vi "Lidar V2 RT Main.vi"() -> ()   [LabVIEW 2013]
uses:
  <vilib>/FPGAPlugInAG/PXIe-7962R/niLvFpga_Open_PXIe-7962R.vi
  <vilib>/rvi/interface/common/dynamic/niFpgaDynamicAddResources.vi
  <vilib>/FPGAPlugInAG/Dynamic/niLvFpga_Abort_Dynamic.vi
  <vilib>/FPGAPlugInAG/Dynamic/niLvFpga_Reset_Dynamic.vi
  <vilib>/FPGAPlugInAG/Dynamic/niLvFpga_Run_Dynamic.vi
  <vilib>/rvi/interface/common/niFpgaWaitOnOcc.vi
  <vilib>/Utility/error.llb/Error Cluster From Error Code.vi
  <vilib>/rvi/errors/niLvFpgaAdjustHostInterfaceError.vi
  <vilib>/FPGAPlugInAG/Dynamic/niLvFpga_Close_Dynamic.vi
  <vilib>/rvi/interface/nirviOpenFPGA/nirviOpenFPGA.xnode
  FPGA Bitfiles/LIDAR Module 5782 V5.9.lvbitx
  <vilib>/rvi/interface/nirviMethod/nirviMethod.xnode
  <vilib>/rvi/interface/nirviReadWriteControl/nirviReadWriteControl.xnode
  <vilib>/rvi/interface/nirviCloseFPGA/nirviCloseFPGA.xnode
  <vilib>/FPGAPlugInAG/Dynamic/niLvFpga_ReadFifo_Dynamic.vi
  <vilib>/rvi/errors/niLvFpgaMergeErrorWithErrorCode.vi
  <vilib>/ptbypt/NI_PtbyPt.lvlib
  <vilib>/Analysis/NI_AALBase.lvlib
  NiFpgaLv.dll
  <vilib>/rvi/interface/Simulation/niFpgaSimulationCallBeginRW.vi
panel:
  in  "MaxStartSample":u8=54
  out "Intensity Map":u32[][](graph)=[[38267, 40863, 43426, 46903, 50379, 49577, 9511, 20052, 7258, 36545, 49622, 30765, 7679, 11446, 11287, 8610], [45519, 42398, 47961, 47044, 51202, 50615, 46477, 39458, 9841, 41698, 52891, 31717, 7088, 8130, 9027, 8119], [48671, 50114, 49333, 52463, 55996, 55598, 55499, 50228, 23748, 32917, 46824, 34677, 16354, 12518, 13710, 14465], [54064, 48927, 52198, 54292, 54548, 47730, 56020, 55390, 37937, 50069, 55178, 34706, 86530, 9874, 15467, 8958], [54127, 52666, 53875, 65066, 101095, 130103, 75733, 59949, 29491, 65502, 50785, 24349, 16198, 8817, 5686, 6636], [63717, 51110, 54640, 82482, 144722, 130520, 117220, 19151, 20018, 18186, 19523, 16677, 18204, 12359, 7312, 6192], [60324, 57984, 72516, 113653, 133185, 141195, 138982, 19785, 13914, 20568, 17572, 18332, 36391, 16559, 8656, 7239], [10675, 84263, 85858, 130204, 147736, 162189, 159832, 21467, 21876, 17164, 11455, 43385, 116640, 15279, 7969, 6867], [37695, 141137, 100147, 149060, 144081, 168934, 167216, 19438, 20260, 21484, 18662, 15530, 119323, 10502, 5990, 5756], [69488, 62058, 50045, 120398, 134387, 151104, 149833, 157001, 47922, 18908, 19123, 19272, 18373, 18944, 18110, 15447], [59157, 62414, 58749, 57578, 60555, 55810, 53103, 60527, 53706, 145306, 42304, 18833, 19783, 8385, 18856, 18720], [64249, 59919, 59597, 60756, 61047, 63017, 64938, 58053, 10510, 155082, 62144, 37988, 7375, 10245, 16147, 15414], [62678, 57333, 55641, 62329, 59085, 64488, 62926, 68318, 5831, 27753, 56193, 49801, 7109, 11185, 14695, 13534], [64860, 57918, 61295, 61918, 64011, 61837, 64216, 68709, 45145, 38007, 52474, 54336, 122862, 23649, 16487, 16877], [64466, 54840, 60724, 63188, 59161, 63167, 61944, 113757, 46296, 65445, 86895, 55833, 117827, 25177, 22545, 24674], [63747, 55429, 56781, 62403, 60957, 62337, 68183, 109145, 46415, 64989, 46515, 60255, 95561, 24349, 18046, 19264], [59827, 54805, 52448, 56788, 59923, 57562, 61463, 61241, 41494, 17316, 22198, 36981, 63082, 17749, 12719, 12336], [55570, 53617, 51599, 51841, 54806, 55615, 59827, 59503, 38863, 55313, 57948, 58576, 79827, 20327, 14840, 15093], [52952, 51728, 52895, 50260, 50904, 54415, 56882, 53800, 42244, 17470, 32064, 64825, 52564, 15197, 14516, 13645], [45412, 46585, 49451, 49892, 46454, 50593, 66473, 70481, 31893, 54244, 80137, 82405, 102857, 102147, 33680, 28535]]
  in  "10thIndexDeb":u8
  in  "ActiveLedIndexDeb":u16
  in  "LedScanDebEn":bool
  out "Numeric":i32=1666
  in  "LaserPower 1":bool=TRUE
  in  "LaserPower 0":bool=TRUE
  out "median":dbl=92741.0 format="%0.2f"
  out "Range Map":u32[][](graph)=[[93610, 93475, 93265, 93026, 92936, 93011, 90522, 93400, 92936, 93355, 93340, 93086, 91182, 91587, 91437, 91437], [93385, 93370, 93250, 93205, 93041, 92936, 92666, 93131, 91976, 93280, 93190, 93250, 92441, 92336, 91811, 91437], [93550, 93445, 93026, 92726, 92576, 92321, 92471, 93385, 93146, 93101, 93086, 93101, 95934, 92681, 86595, 86340], [93655, 93595, 93071, 92681, 92531, 89158, 92546, 93325, 92936, 92996, 93190, 93340, 93280, 88993, 86550, 88094], [93460, 93280, 93026, 86940, 86625, 86715, 86745, 91841, 91976, 92306, 93295, 92936, 86760, 86610, 89938, 89938], [93190, 93250, 86565, 86505, 86475, 86370, 86325, 86520, 86505, 86760, 86415, 86580, 86580, 92741, 91437, 89938], [93325, 93190, 86730, 86535, 86445, 86475, 86475, 86670, 86550, 86565, 86430, 86625, 93985, 92756, 90897, 89938], [95829, 86685, 86550, 86460, 86475, 86520, 86580, 86535, 86430, 86580, 92936, 93131, 93175, 92621, 90477, 89938], [93101, 86400, 86160, 86145, 86235, 86280, 86130, 86490, 86385, 86445, 86580, 86940, 93011, 86835, 90118, 89938], [93026, 92861, 92756, 86370, 86265, 86160, 86160, 86115, 86400, 86460, 86400, 86505, 86625, 86490, 86535, 86565], [93220, 93190, 93056, 92771, 92576, 92486, 92501, 92861, 86220, 86070, 86280, 86565, 86550, 88694, 86565, 86460], [93146, 93235, 92786, 92621, 92606, 92621, 92726, 92801, 90537, 92336, 92711, 92726, 96158, 91437, 91317, 91047], [92891, 92771, 92771, 92756, 92801, 92816, 92666, 92696, 91437, 92651, 92816, 92711, 93101, 91856, 91811, 91781], [92936, 92936, 93041, 93011, 92996, 92936, 92936, 92936, 92486, 92936, 92936, 92936, 93041, 92771, 92306, 92126], [93041, 93131, 93026, 92726, 92681, 92666, 92621, 92351, 91856, 91796, 92606, 92756, 92936, 92681, 91871, 91751], [93175, 93161, 92846, 92786, 92726, 92861, 92636, 92216, 91796, 91826, 92816, 92816, 92756, 92441, 91437, 91602], [92936, 92741, 92726, 92756, 92936, 92771, 92741, 92711, 91811, 92591, 92711, 92681, 92726, 92351, 91437, 91766], [92771, 92846, 92861, 92936, 92771, 92711, 92771, 92786, 92111, 92591, 92666, 92786, 92936, 92591, 92216, 91677], [93071, 93086, 93041, 92816, 92741, 92786, 92936, 93056, 91871, 92441, 92606, 92831, 92936, 92516, 91437, 91212], [93026, 92936, 92831, 92711, 92756, 92936, 92426, 92351, 90597, 90612, 90642, 90642, 90447, 90402, 90238, 90223]]
  in  "PulseUpClck":u16=4
  in  "PulseWaitClck":u16=30
  in  "Devider":u8=1
  in  "ScanFormat":enum16{"1PulsePerLed", "FullScanPerLed"}(ring)=enum."FullScanPerLed"
  in  "Freq [Mhz]":dbl=100000000.0 format="%#_6p"
  out "error out":errorcluster
  out "standard deviation":dbl=2806.7231162507614 format="%0.5f"
  out "Coarse":dbl
  out "Fine":dbl
  in  "empty graph data":bool
  out "hi(x) 2":i32[][](graph)
  out "hi(x)":i32[](array[numeric])
  out "interval":u32=4
  in  "y":dbl=57.0
  out "Range":dbl=0.4861031988439848 format="%#.2f"
  out "Distance":dbl=88993.39115730001 format="%#.4f"
  out "mean":dbl=57.486103198843985 format="%0.2f"
  out "Fine":u16[](array[numeric])=[88, 76, 70, 116, 105, 79, 74, 115, 111, 107, 100, 88, 86, 100, 100, 134, 110, 60, 83, 137]
  out "Coarse":u16[](array[numeric])=[57, 57, 62, 61, 61, 57, 57, 63, 61, 61, 61, 61, 61, 61, 61, 59, 60, 61, 61, 58]
  in  "stop":bool=TRUE
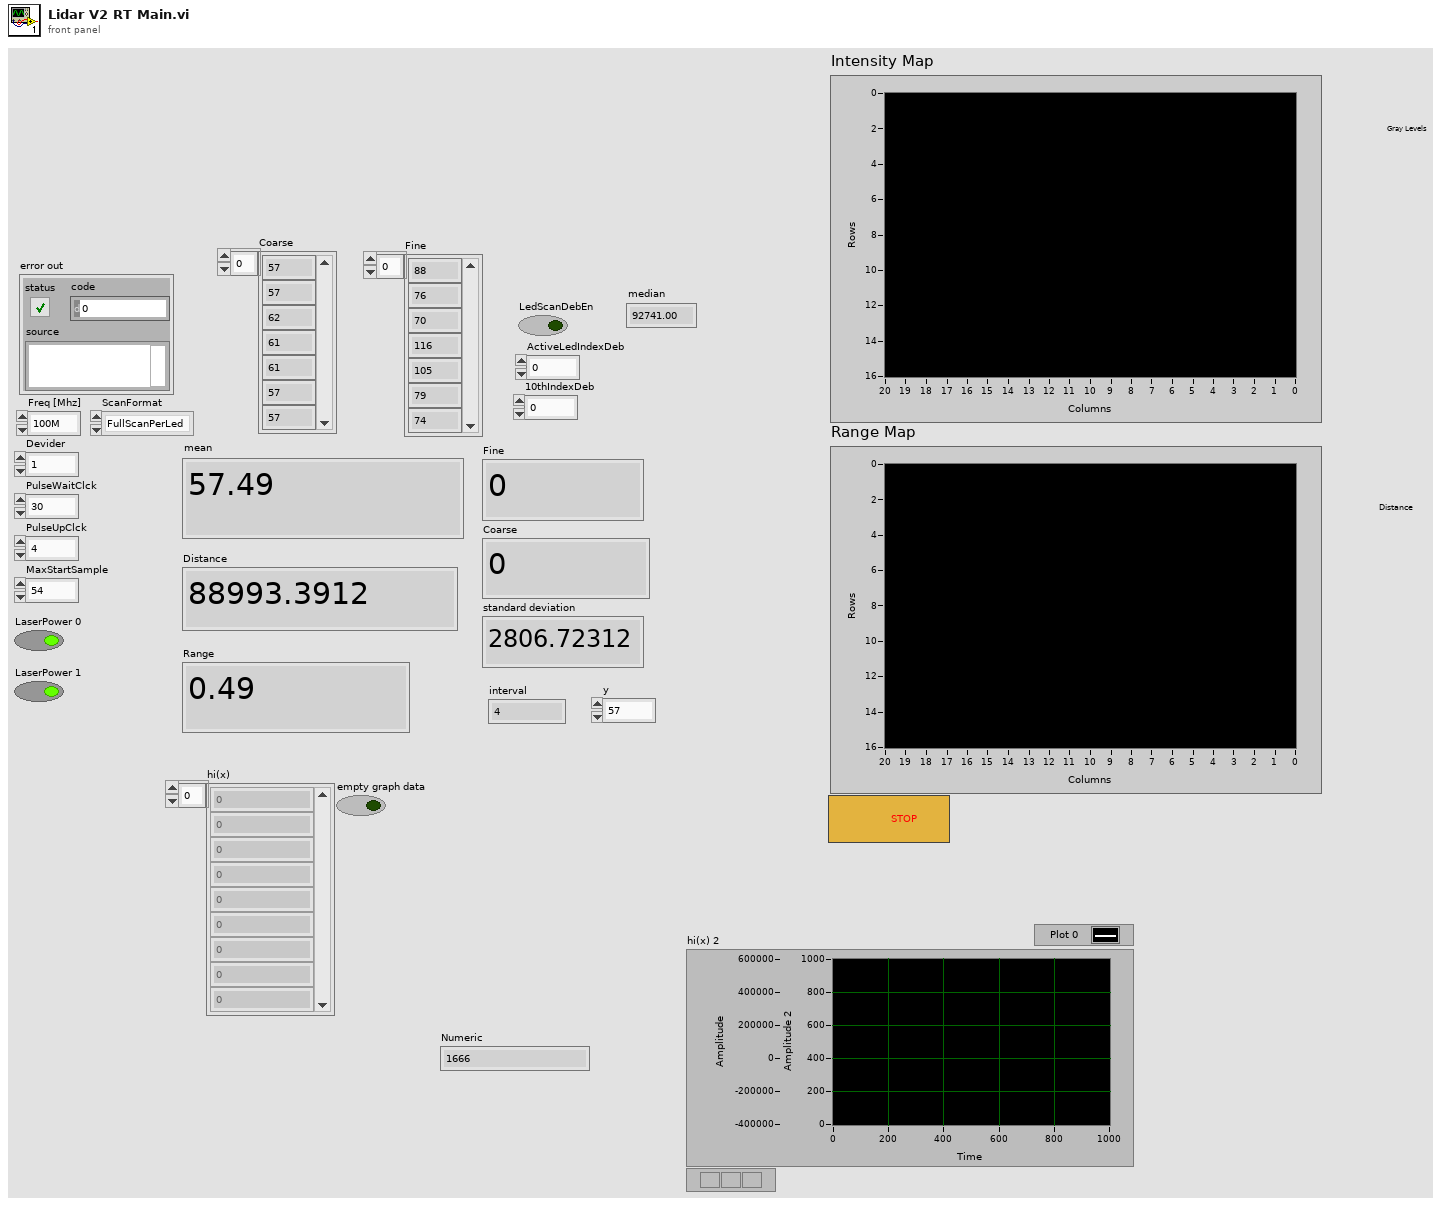
[diagram p1: front panel]
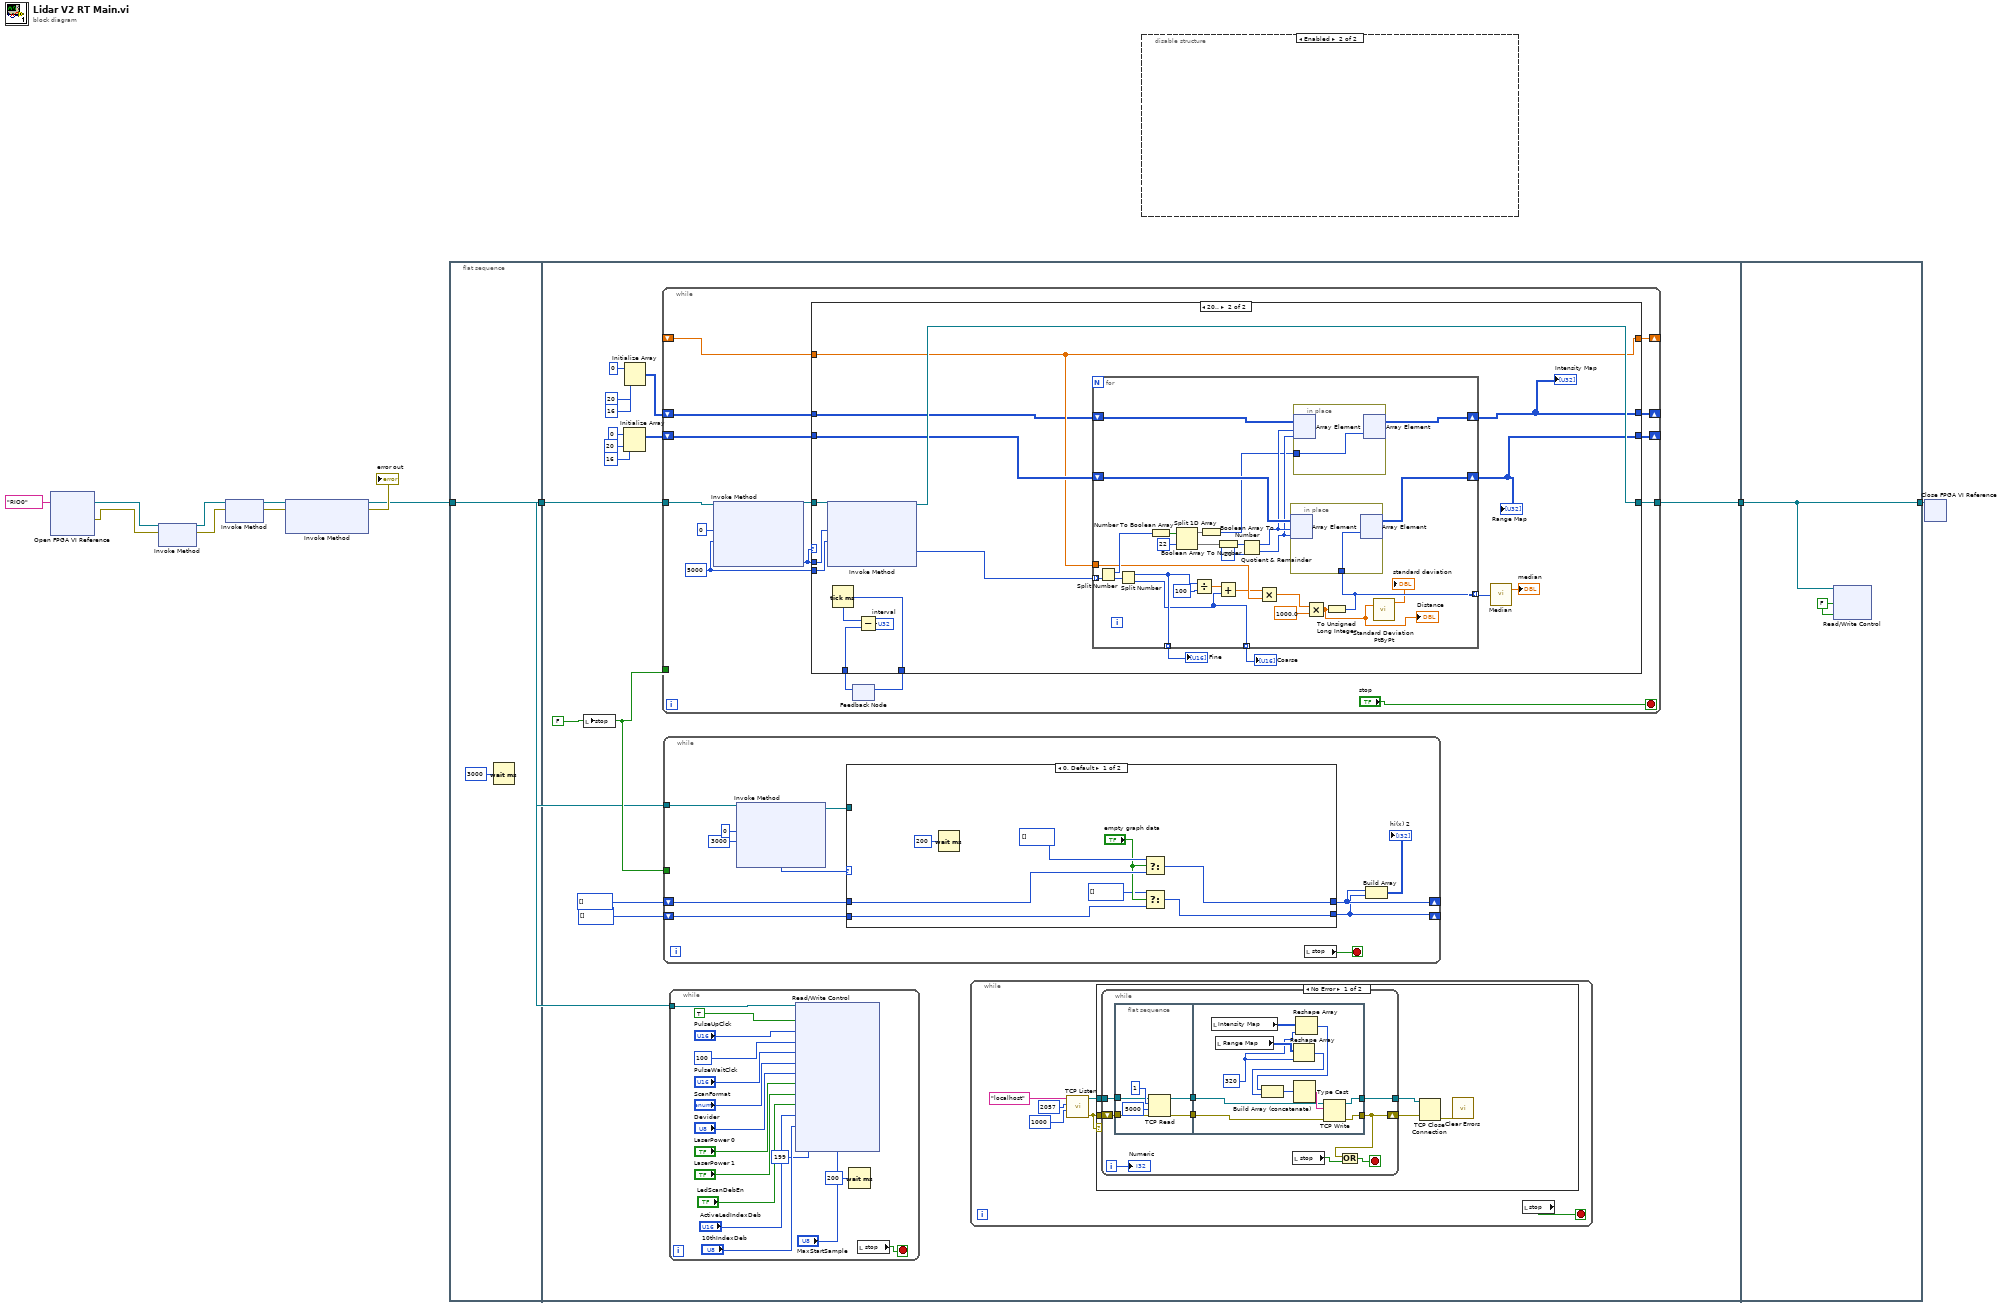
[diagram p0: block diagram]
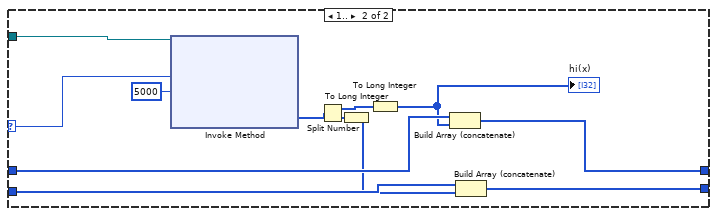
[diagram p3: hidden frame]
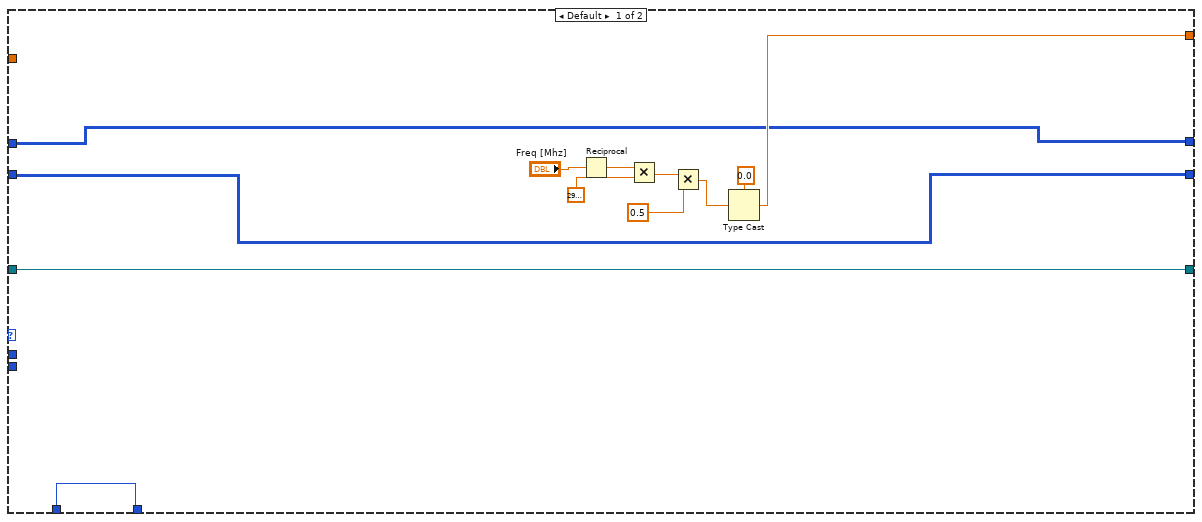
[diagram p4: hidden frame]
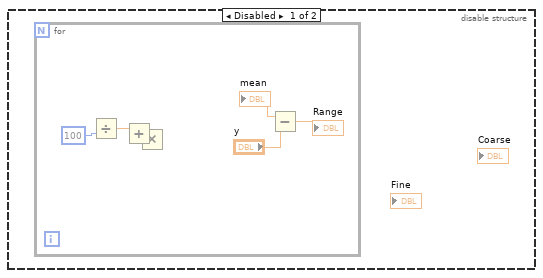
[diagram p5: hidden frame]
diagram:
  n1 = xnode "Open FPGA VI Reference"("resource name"=tag "RIO0") -> ("FPGA VI Reference Out"=w4:refnum<k20>, "error out"=w2:errorcluster)  [unwired: 1 in]
  n2 = xnode "Invoke Method"("FPGA VI Reference In"=w4, "error in"=w2) -> ("FPGA VI Reference Out"=w3:refnum<k20>, "error out"=w1:errorcluster)
  n3 = xnode "Invoke Method"("FPGA VI Reference In"=w3, "error in"=w1) -> ("FPGA VI Reference Out"=w10:refnum<k20>, "error out"=w9:errorcluster)
  n4 = xnode "Invoke Method"("FPGA VI Reference In"=w10, "error in"=w9) -> ("FPGA VI Reference Out"=w7:refnum<k20>, "error out"=→"error out":errorcluster)  [unwired: 1 in]
  n5 = flat-sequence {
    tunnel: w7 -> [w14]
    tunnel: [w14] -> w6
    tunnel: w6 -> [w23]
    tunnel: [w27] -> w5
    tunnel: [w186] -> w11
    tunnel: w5 -> [w186]
    frame #0 {
      n6 = Wait (ms)(milliseconds to wait=u32 3000) -> ()  [unwired: 1 out]
    }
    frame #1 {
      w26 = FALSE ("stop")
      n7 = local write "stop"(w26) -> ()
      n8 = Initialize Array(u32 0 ("element"), 20 ("dimension size"), 16 ("dimension size")) -> (w19:u32[][])
      n9 = Initialize Array(u32 0 ("element"), 20 ("dimension size"), 16 ("dimension size")) -> (w15:u32[][])
      n10 = while {
        tunnel: w23 -> [w126]
        tunnel: [w121] -> w27
        tunnel: w26 -> [_]
        shift-right: [w117] -> _
        shift-left: _ -> [w116]
        shift-right: [w114] -> _
        shift-left: w19 -> [w115]
        shift-right: [w112] -> _
        shift-left: w15 -> [w113]
        stop <- "stop" stop-if-true
        w123 = 5000 ("Timeout (ms)")
        n11 = xnode "Invoke Method"("FPGA VI Reference In"=w126, "Number of Elements"=u32 0, "Timeout (ms)"=w123) -> ("FPGA VI Reference Out"=w124:refnum<k20>, "Elements Remaining"=w120:u32)  [unwired: 1 in, 2 out]
        n12 = feedback #1() -> (w118:u32)  [unwired: 1 in]
        n13 = case shown="20.." w120 {
          tunnel: w124 -> [w138 w155]
          tunnel: w120 -> [_ w154]
          tunnel: w123 -> [_ w153]
          tunnel: [w138 w151] -> w121
          tunnel: [w137 w150] -> w119
          tunnel: w118 -> [w137 w149]
          tunnel: [w129 w146] -> w117
          tunnel: w116 -> [_ w146]
          tunnel: w115 -> [w128 w147]
          tunnel: [w128 w145] -> w114
          tunnel: w113 -> [w127 w140]
          tunnel: [w127 w139] -> w112
          frame Default {
            n14 = Reciprocal(x="Freq [Mhz]") -> (1/x=w136:dbl)
            n15 = Multiply(x=w136, y=dbl[unit] 299792458.0) -> (x*y=w133:dbl[unit])
            n16 = Multiply(x=w133, y=dbl[unit] 0.5) -> (x*y=w130:dbl[unit])
            n17 = Type Cast(type=0.0 ("y"), x=w130) -> (*(type *) &x=w129:dbl)
          }
          frame 20.. {
            n18 = xnode "Invoke Method"("FPGA VI Reference In"=w155, "Number of Elements"=w154, "Timeout (ms)"=w153) -> ("FPGA VI Reference Out"=w151:refnum<k20>, "Data"=w152:u64[])  [unwired: 1 in, 2 out]
            n19 = Tick Count (ms)() -> (millisecond timer value=w150:u32)
            n20 = Subtract(x=w150, y=w149) -> (x-y=→"interval":u32)
            n21 = for {
              tunnel: w152 -> [w182] mode=indexing
              shift-right: [w178] -> w145
              shift-left: w147 -> [w179]
              tunnel: w146 -> [w177]
              tunnel: [w176] -> w144 mode=indexing
              tunnel: [w175] -> w142 mode=indexing
              tunnel: [w172] -> w141 mode=indexing
              shift-right: [w173] -> w139
              shift-left: w140 -> [w174]
              n22 = Split Number(x=w182) -> (hi(x)=w180:u32, lo(x)=w181:u32)
              n23 = Split Number(x=w181) -> (hi(x)=w175:u16, lo(x)=w172:u16)
              n24 = Number To Boolean Array(number=w180) -> (Boolean array=w171:bool[])
              n25 = Split 1D Array(array=w171, index=22) -> (first subarray=w157:bool[], second subarray=w169:bool[])
              n26 = Divide(x=w175, y=u16 100) -> (x/y=w165:dbl)
              n27 = Boolean Array To Number(Boolean array=w157) -> (number=w156:u32)
              n28 = Add(x=w165, y=w172) -> (x+y=w166:dbl)
              n29 = Boolean Array To Number(Boolean array=w169) -> (number=w168:u32)
              n30 = Quotient & Remainder(x=w168, y=u32 20) -> (x-y*floor(x/y)=w159:u32, floor(x/y)=w158:u32)
              n31 = Multiply(x=w166, y=w177) -> (x*y=w162:dbl)
              n32 = in-place {
                in-place-border: w156 -> [w183]
                n33 = in-place-array #2(w174, w159, w158) -> ()  [unwired: 1 out]
                n34 = in-place-array #2(w183) -> (w173:u32[][])  [unwired: 2 out]
              }
              n35 = Multiply(x=w162, y=1000.0) -> (x*y=w160:dbl)
              "Distance" <- w160
              n36 = To Unsigned Long Integer(number=w160) -> (unsigned 32bit integer=w176:u32)
              n37 = in-place {
                in-place-border: w176 -> [w184]
                n38 = in-place-array #3(w179, w159, w158) -> ()  [unwired: 1 out]
                n39 = in-place-array #3(w184) -> (w178:u32[][])  [unwired: 2 out]
              }
              n40 = call <vilib>:"Standard Deviation PtByPt.vi"("x"=w160) -> ("standard deviation"=→"standard deviation":dbl)  [unwired: 2 in, 2 out]
            }
            "Coarse" <- w141
            "Fine" <- w142
            "Range Map" <- w145
            "Intensity Map" <- w139
            n41 = call <vilib>:"Median.vi"("X"=w144) -> ("median"=→"median":dbl)  [unwired: 1 out]
          }
        }
        n42 = feedback-in #1(w119) -> ()
      }
      n43 = while {
        tunnel: w23 -> [w91]
        tunnel: w26 -> [_]
        shift-right: [w83] -> _
        shift-left: i32[] [] -> [w85]
        shift-right: [w82] -> _
        shift-left: i32[] [] -> [w84]
        stop <- w86 stop-if-true
        n44 = xnode "Invoke Method"("FPGA VI Reference In"=w91, "Number of Elements"=u32 0, "Timeout (ms)"=3000) -> ("FPGA VI Reference Out"=w90:refnum<k20>, "Elements Remaining"=w87:u32)  [unwired: 1 in, 2 out]
        n45 = case shown="0, Default" w87 {
          selector: w87 -> [_ w110]
          tunnel: w90 -> [_ w111]
          tunnel: [w97 w105] -> w83
          tunnel: w85 -> [w99 w107]
          tunnel: [w94 w102] -> w82
          tunnel: w84 -> [w95 w101]
          frame 0, Default {
            n46 = Wait (ms)(milliseconds to wait=u32 200) -> ()  [unwired: 1 out]
            n47 = Select(t=i32[] [] ("f"), s="empty graph data", f=w99) -> (s? t:f=w97:i32[])
            n48 = Select(t=i32[] [], s="empty graph data", f=w95) -> (s? t:f=w94:i32[])
          }
          frame 1.. {
            n49 = xnode "Invoke Method"("FPGA VI Reference In"=w111, "Number of Elements"=w110, "Timeout (ms)"=5000) -> ("Data"=w108:u64[])  [unwired: 1 in, 3 out]
            n50 = Split Number(x=w108) -> (hi(x)=w106:u32[], lo(x)=w103:u32[])
            n51 = To Long Integer(number=w103) -> (32bit integer=w100:i32[])
            n52 = To Long Integer(number=w106) -> (32bit integer=w104:i32[])
            "hi(x)" <- w104
            n53 = Build Array (concatenate)(w107, w104) -> (w105:i32[])
            n54 = Build Array (concatenate)(w101, w100) -> (w102:i32[])
          }
        }
        n55 = local read "stop"() -> (w86:bool)
        n56 = Build Array(w83, w82) -> (→"hi(x) 2":i32[][])
      }
      n57 = while {
        tunnel: w23 -> [w75]
        stop <- w74 stop-if-true
        n58 = xnode "Read/Write Control"("FPGA VI Reference In"=w75, "SamplingEnable"=TRUE, "PulseUpClck"="PulseUpClck", "SampPerPulse"=u16 100, "PulseWaitClck"="PulseWaitClck", "ScanFormat"="ScanFormat", "Devider"="Devider", "PFI2"="LaserPower 0", "PFI3"="LaserPower 1", "LedScanDebEn"="LedScanDebEn", "ActiveLedIndexDeb"="ActiveLedIndexDeb", "10thIndexDeb"="10thIndexDeb", "MaxStartSample"="MaxStartSample", "PulsePerLed"=i16 199) -> ()  [unwired: 1 in, 2 out]
        n59 = Wait (ms)(milliseconds to wait=u32 200) -> ()  [unwired: 1 out]
        n60 = local read "stop"() -> (w74:bool)
      }
      n61 = while {
        stop <- w29 stop-if-true
        n62 = call <vilib>:"TCP Listen.vi"("timeout ms (wait forever: -1)"=1000, "port"=u16 2057, "service name"="localhost" ("address")) -> ("error out"=w28:errorcluster, "connection ID"=w33:refnum<k5>)  [unwired: 4 in, 3 out]
        n63 = case shown="No Error" w28 {
          tunnel: w28 -> [w36 _]
          tunnel: w33 -> [w35 _]
          frame No Error {
            n64 = while {
              tunnel: w35 -> [w47]
              tunnel: [w41] -> w37
              shift-right: [w39] -> w38
              shift-left: w36 -> [w46]
              i -> [w44]
              stop <- w40 stop-if-true
              n65 = flat-sequence {
                tunnel: w47 -> [w50]
                tunnel: w46 -> [w49]
                tunnel: [w53] -> w43
                tunnel: [w52] -> w42
                tunnel: w43 -> [w62]
                tunnel: w42 -> [w61]
                tunnel: [w60] -> w41
                tunnel: [w59] -> w39
                frame #0 {
                  n66 = TCP Read(connection ID=w50, bytes to read=1, error in (no error)=w49, 9:5000 ("timeout ms (25000)")) -> (connection ID out=w53:refnum<k5>, error out=w52:errorcluster)  [unwired: 1 in, 1 out]
                }
                frame #1 {
                  w57 = 320 ("dimension size")
                  n67 = local read "Intensity Map"() -> (w58:u32[][])
                  n68 = local read "Range Map"() -> (w64:u32[][])
                  n69 = Reshape Array(w64, w57) -> (w55:u32[])
                  n70 = Reshape Array(w58, w57) -> (w56:u32[])
                  n71 = Build Array (concatenate)(w56, w55) -> (w54:u32[])
                  n72 = Type Cast(x=w54) -> (*(type *) &x=w63:string)  [unwired: 1 in]
                  n73 = TCP Write(connection ID=w62, data in=w63, error in (no error)=w61) -> (connection ID out=w60:refnum<k5>, error out=w59:errorcluster)  [unwired: 1 in, 1 out]
                }
              }
              n74 = local read "stop"() -> (w45:bool)
              n75 = Or(x=w39, y=w45) -> (x .or. y?=w40:bool)
              "Numeric" <- w44
            }
            n76 = TCP Close Connection(connection ID=w37, error in (no error)=w38) -> (error out=w34:errorcluster)  [unwired: 1 in, 1 out]
            n77 = call <vilib>:"Clear Errors.vi"("error in (no error)"=w34) -> ()  [unwired: 6 in, 1 out]
          }
          frame Error {
          }
        }
        n78 = local read "stop"() -> (w29:bool)
      }
    }
    frame #2 {
      w185 = FALSE ("PFI2")
      n79 = xnode "Read/Write Control"("FPGA VI Reference In"=w186, "PFI2"=w185, "PFI3"=w185) -> ()  [unwired: 1 in, 2 out]
    }
  }
  n80 = disable-structure shown="Enabled" {
    frame Disabled {
      n81 = for {
        n82 = Divide(y=u16 100) -> (x/y=w192:dbl)  [unwired: 1 in]
        n83 = Add(x=w192) -> (x+y=w191:dbl)  [unwired: 1 in]
        n84 = Multiply(x=w191) -> (x*y=w187:dbl)  [unwired: 1 in]
        n85 = Subtract(x="mean", y="y") -> (x-y=→"Range":dbl)
      }
    }
    frame Enabled {
    }
  }
  n86 = xnode "Close FPGA VI Reference"("FPGA VI Reference In"=w11) -> ()  [unwired: 1 in, 1 out]
